vi "Feedback from APD.vi"(7 "Set Point":dbl, 8 "error in (no error)":errorcluster, 9 "Piezo Message Queue":refnum<queue>, 10 "Piezo Readout":refnum<notifier>, 11 "APD Position Data":refnum<notifier>) -> (0 "error out":errorcluster)   [LabVIEW 2013, in "Feedback.lvlib"]
uses:
  Feedback.lvlib
  support/Message Queue/Message Cluster.ctl
  Piezo/Piezo display.ctl
  support/Message Queue/Message Queue.lvlib
  Desktop/Simon Labview/Piezo.lvlib
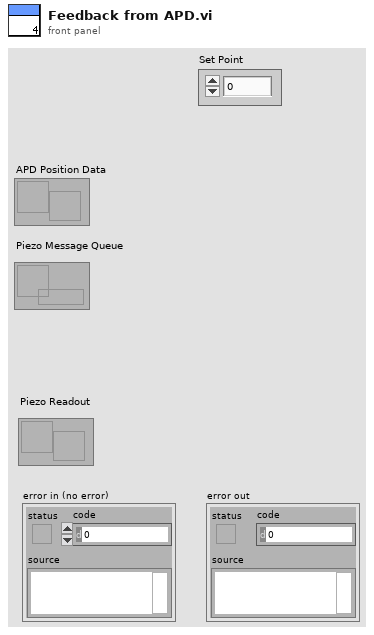
[diagram p1: front panel]
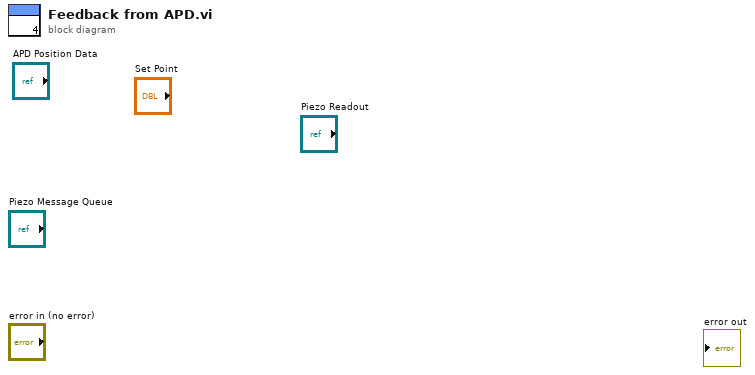
[diagram p0: block diagram]
diagram:
